vi "bats.filter.runFpgaTests.vi"() -> ()   [LabVIEW 2020]
panel:
  out "CRC32 Passed":bool
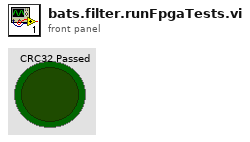
[diagram p1: front panel]
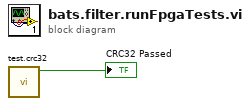
[diagram p0: block diagram]
diagram:
  n1 = call "test.crc32.vi"() -> ("All Passed"=→"CRC32 Passed":bool)  [unwired: 11 in]
